vi "Client Closed.vi"(8 "error in (no error)":errorcluster, 10 "WS Client":refnum<class "WebSocket Client.lvclass">, 11 "WebSocket Manager in":refnum<class "WebSocket Manager.lvclass">) -> (0 "error out":errorcluster)   [LabVIEW 2020, in "HTTP Server.lvlib" / "WebSocket Manager.lvclass"]
uses:
  WebSocket Manager.lvclass
  WebSocket Client/WebSocket Client.lvclass
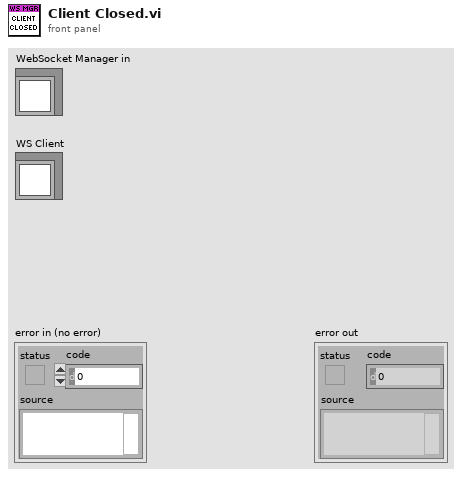
[diagram p1: front panel]
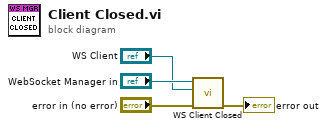
[diagram p0: block diagram]
diagram:
  n1 = call-dynamic "WS Client Closed.vi"("error in (no error)"="error in (no error)", "WS Client"="WS Client", "WebSocket Manager in"="WebSocket Manager in") -> ("error out"=→"error out":errorcluster)  [unwired: 8 in]
